vi "Module Type.vi"(11 "DemoClass in":refnum<class "DemoClass.lvclass">) -> (2 "Module Type":string)   [LabVIEW 2020, in "VolatusScratch.lvlib" / "DemoClass.lvclass"]
uses:
  DemoClass.lvclass
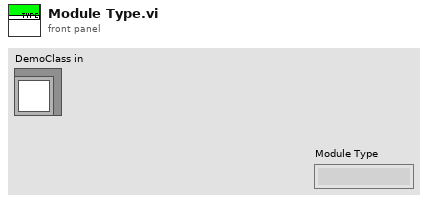
[diagram p1: front panel]
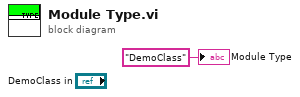
[diagram p0: block diagram]
diagram:
  "Module Type" <- "DemoClass" ("Module Type")
